vi "Kei237_Read_I_Command.vi"(1 "error in":errorcluster, 2 "GPIB":string) -> (0 "error out":errorcluster)   [LabVIEW 2009]
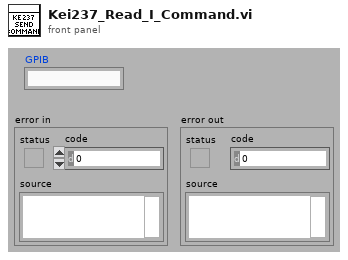
[diagram p1: front panel]
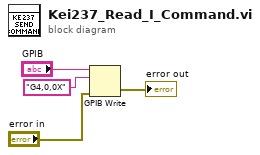
[diagram p0: block diagram]
diagram:
  n1 = GPIB Write(0:"GPIB", 1:"G4,0,0X" ("data"), 3:"error in") -> (6:→"error out":errorcluster)  [unwired: 2 in, 1 out]
